vi "GetUserDefinedAssetsDirectory.vi"(8 "Error In":errorcluster) -> (0 "Error Out":errorcluster, 3 "User Defined Assets Directory":path)   [LabVIEW 2018, in "Asset.lvclass"]
uses:
  Asset/Asset.lvclass
  <vilib>/Utility/sysdir.llb/System Directory Type.ctl
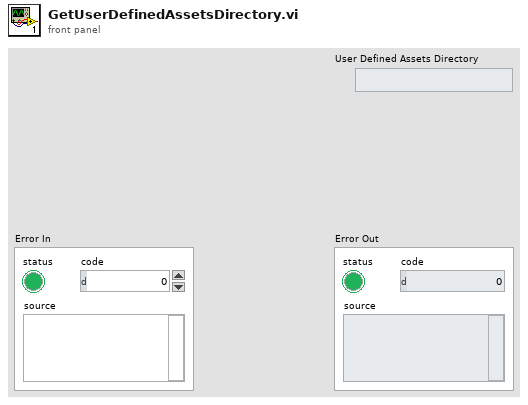
[diagram p1: front panel]
types:
  T1 = typedef "System Directory Type.ctl" = i32
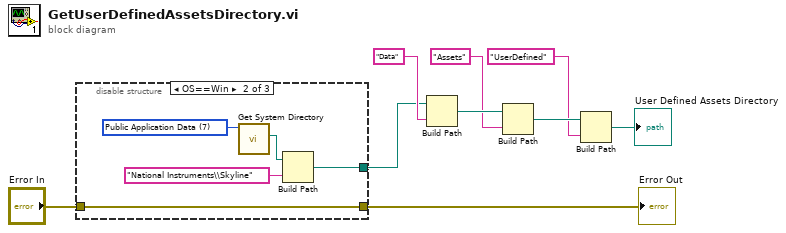
[diagram p0: block diagram]
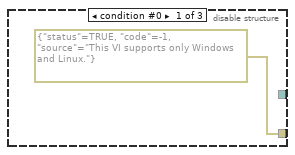
[diagram p2: hidden frame]
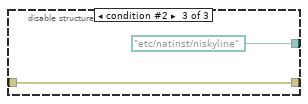
[diagram p3: hidden frame]
diagram:
  n1 = disable-structure shown="OS==Win" {
    disable-tunnel: [_ w12 path "/etc/natinst/niskyline" ("base path")] -> w2
    disable-tunnel: "Error In" -> [_ w11 w16]
    disable-tunnel: [errorcluster {"status"=TRUE, "code"=-1, "source"="This VI supports only Windows and Linux."} ("error constant") w11 w16] -> w8
    frame condition #0 {
    }
    frame condition #1 (active) {
      w15 = T1 7 items=["User Home"=0, "User Desktop"=1, "User Documents"=2, "User Application Data"=3, "User Preferences"=4, "User Temporary"=5, "Public Documents"=6, "Public Application Data"=7, "Public Preferences"=8, "Public Cache"=13, "System Core Libraries"=9, "System Installed Libraries"=10, "Application Files"=11, "Boot Volume Root"=12] ("system directory type")
      n2 = call <vilib>:"Get System Directory.vi"("system directory type"=w15) -> ("system directory"=w14:path)  [unwired: 10 in]
      n3 = Build Path(base path=w14, name or relative path="National Instruments\\Skyline") -> (appended path=w12:path)
    }
    frame condition #2 {
    }
  }
  "Error Out" <- w8
  n4 = Build Path(base path=w2, name or relative path="Data") -> (appended path=w6:path)
  n5 = Build Path(base path=w6, name or relative path="Assets") -> (appended path=w4:path)
  n6 = Build Path(base path=w4, name or relative path="UserDefined") -> (appended path=→"User Defined Assets Directory":path)
